vi "create.vi"(8 "error in (no error)":errorcluster, 10 "FASettings":T1, 11 "FAILCFactory in":refnum<class "FAILCFactory.lvclass">) -> (0 "error out":errorcluster, 2 "ForceActuator":refnum<class "FAILC.lvclass">, 3 "FAILCFactory out":refnum<class "FAILCFactory.lvclass">)   [LabVIEW 2016, in "RTFAILC.lvlib" / "FAILCFactory.lvclass"]
uses:
  FAILCFactory.lvclass
  DataTypes/FASettings.ctl
  Common_RT_ILC/DataTypes/ILCSettings.ctl
  DataTypes/FATypes.ctl
  FAILC/FAILC.lvclass
  SAAILC/SAAILC.lvclass
  D:/Code/ts_FAMT/Common_RT_FAILC/FAILC/FAILC.lvclass
  D:/Code/ts_FAMT/Common_RT_ILC/ILC/ILC.lvclass
  DataTypes/FAData.ctl
  DataTypes/FAConstants.ctl
  DataTypes/FACommand.ctl
  DataTypes/FAPID.ctl
  DataTypes/FATelemetry.ctl
  DataTypes/FAResponses.ctl
  Common_RT_Modbus/DataTypes/ExceptionCodes.ctl
  Common_RT_ILC/ILCFactory/ILCFactory.lvclass
  FAILC/FAILC.lvclass/FAILC.ctl
  DAAILC/DAAILC.lvclass
  RTFAILC.lvlib
  Common_RT_Modbus/RTModbus.lvlib
  Common_RT_ILC/RTILC.lvlib
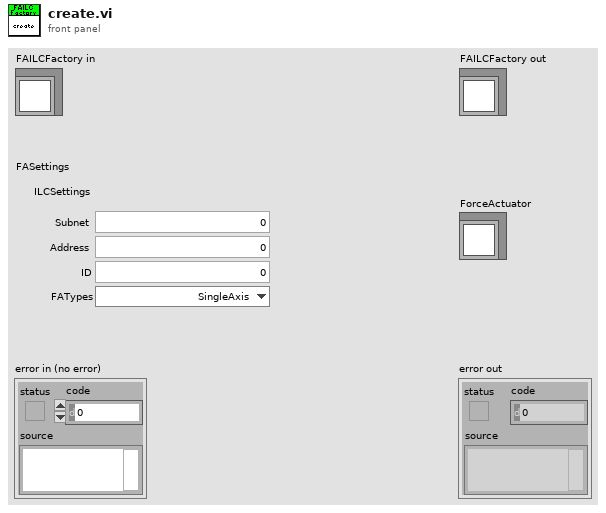
[diagram p1: front panel]
types:
  T1 = typedef "RTFAILC.lvlib/FASettings.ctl" = cluster{"ILCSettings":T2, "ID":i16, "FATypes":T3}
  T2 = typedef "RTILC.lvlib/ILCSettings.ctl" = cluster{"Subnet":u8, "Address":u8}
  T3 = typedef "RTFAILC.lvlib/FATypes.ctl" = enum16{"SingleAxis", "LateralDualAxis", "CrossLateralDualAxis"}
  T4 = typedef "RTFAILC.lvlib/FAData.ctl" = cluster{"FAConstants":T5, "FACommand":T6, "FATelemetry":T8, "FAResponses":T9}
  T5 = typedef "RTFAILC.lvlib/FAConstants.ctl" = cluster{"ID":i16}
  T6 = typedef "RTFAILC.lvlib/FACommand.ctl" = cluster{"AxialSetPoint":i32, "LateralSetPoint":i32, "PressureServoValveSettings":T7, "BoosterValveSettings":T7}
  T7 = typedef "RTFAILC.lvlib/FAPID.ctl" = cluster{"Kp":sgl, "Ki":sgl, "Kd":sgl, "Kf":sgl}
  T8 = typedef "RTFAILC.lvlib/FATelemetry.ctl" = cluster{"ILCFault":bool, "BroadcastCounter":u8, "AxialLoadCellForce":sgl, "LateralLoadCellForce":sgl, "AxialPressure":T7, "AxialTurbo":T7, "LateralPressure":T7, "LateralTurbo":T7}
  T9 = typedef "RTFAILC.lvlib/FAResponses.ctl" = cluster{"PIDParameters":T10, "ReadPIDParameters":T10, "SetForce":T10, "ForceAndStatus":T10}
  T10 = typedef "RTModbus.lvlib/ExceptionCodes.ctl" = u16
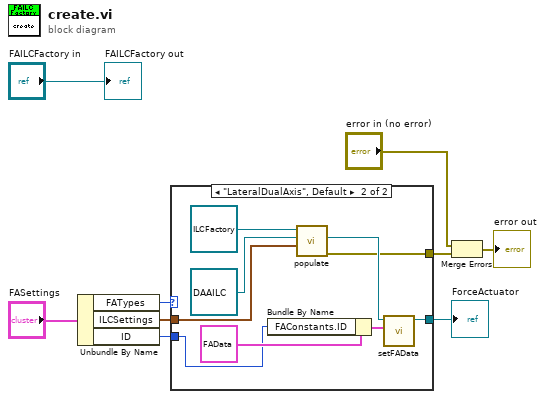
[diagram p0: block diagram]
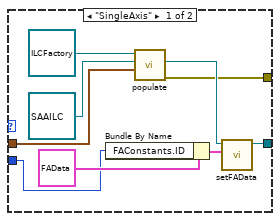
[diagram p2: hidden frame]
diagram:
  n1 = Unbundle By Name("FASettings") -> ("FATypes"=w8:T3, "ILCSettings"=w7:T2, "ID"=w6:i16)
  n2 = case shown="\"LateralDualAxis\", Default" w8 {
    tunnel: w7 -> [w15 w25]
    tunnel: w6 -> [w12 w22]
    tunnel: [w11 w21] -> w5
    tunnel: [w10 w20] -> w4
    frame "SingleAxis" {
      n3 = Bundle By Name(cluster=T4 {"FAConstants"={"ID"=0}, "FACommand"={"AxialSetPoint"=0, "LateralSetPoint"=0, "PressureServoValveSettings"={"Kp"=0.0, "Ki"=0.0, "Kd"=0.0, "Kf"=0.0}, "BoosterValveSettings"={"Kp"=0.0, "Ki"=0.0, "Kd"=0.0, "Kf"=0.0}}, "FATelemetry"={"ILCFault"=FALSE, "BroadcastCounter"=0, "AxialLoadCellForce"=0.0, "LateralLoadCellForce"=0.0, "AxialPressure"={"Kp"=0.0, "Ki"=0.0, "Kd"=0.0, "Kf"=0.0}, "AxialTurbo"={"Kp"=0.0, "Ki"=0.0, "Kd"=0.0, "Kf"=0.0}, "LateralPressure"={"Kp"=0.0, "Ki"=0.0, "Kd"=0.0, "Kf"=0.0}, "LateralTurbo"={"Kp"=0.0, "Ki"=0.0, "Kd"=0.0, "Kf"=0.0}}, "FAResponses"={"PIDParameters"=0, "ReadPIDParameters"=0, "SetForce"=0, "ForceAndStatus"=0}} ("FAData"), "FAConstants.ID"=w12) -> (w13:T4)
      n4 = call "populate.vi"("Settings"=w15, "ILC in"=refnum<class "SAAILC.lvclass"> refnum ("RTFAILC.lvlib:SAAILC.lvclass"), "ILCFactory in"=refnum<class "ILCFactory.lvclass"> refnum ("RTILC.lvlib:ILCFactory.lvclass")) -> ("error out"=w10:errorcluster, "ILC out"=w14:refnum<class "SAAILC.lvclass">)  [unwired: 6 in, 1 out]
      n5 = call "setFAData.vi"("FAData"=w13, "FAILC in"=w14) -> ("FAILC out"=w11:refnum<class "SAAILC.lvclass">)  [unwired: 9 in]
    }
    frame "LateralDualAxis", Default {
      n6 = Bundle By Name(cluster=T4 {"FAConstants"={"ID"=0}, "FACommand"={"AxialSetPoint"=0, "LateralSetPoint"=0, "PressureServoValveSettings"={"Kp"=0.0, "Ki"=0.0, "Kd"=0.0, "Kf"=0.0}, "BoosterValveSettings"={"Kp"=0.0, "Ki"=0.0, "Kd"=0.0, "Kf"=0.0}}, "FATelemetry"={"ILCFault"=FALSE, "BroadcastCounter"=0, "AxialLoadCellForce"=0.0, "LateralLoadCellForce"=0.0, "AxialPressure"={"Kp"=0.0, "Ki"=0.0, "Kd"=0.0, "Kf"=0.0}, "AxialTurbo"={"Kp"=0.0, "Ki"=0.0, "Kd"=0.0, "Kf"=0.0}, "LateralPressure"={"Kp"=0.0, "Ki"=0.0, "Kd"=0.0, "Kf"=0.0}, "LateralTurbo"={"Kp"=0.0, "Ki"=0.0, "Kd"=0.0, "Kf"=0.0}}, "FAResponses"={"PIDParameters"=0, "ReadPIDParameters"=0, "SetForce"=0, "ForceAndStatus"=0}} ("FAData"), "FAConstants.ID"=w22) -> (w23:T4)
      n7 = call "populate.vi"("Settings"=w25, "ILC in"=refnum<class "DAAILC.lvclass"> refnum ("RTFAILC.lvlib:DAAILC.lvclass"), "ILCFactory in"=refnum<class "ILCFactory.lvclass"> refnum ("RTILC.lvlib:ILCFactory.lvclass")) -> ("error out"=w20:errorcluster, "ILC out"=w24:refnum<class "DAAILC.lvclass">)  [unwired: 6 in, 1 out]
      n8 = call "setFAData.vi"("FAData"=w23, "FAILC in"=w24) -> ("FAILC out"=w21:refnum<class "DAAILC.lvclass">)  [unwired: 9 in]
    }
  }
  "ForceActuator" <- w5
  n9 = Merge Errors("error in (no error)", w4) -> (→"error out":errorcluster)
  "FAILCFactory out" <- "FAILCFactory in"
